vi "saltgenerator.vi"(11 "Numeric":i32) -> (3 "string":string)   [LabVIEW 2013]
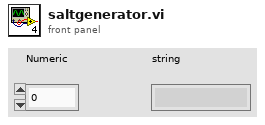
[diagram p1: front panel]
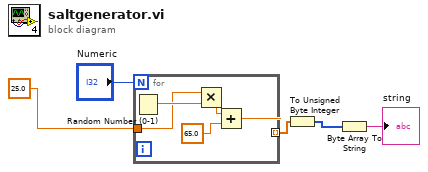
[diagram p0: block diagram]
diagram:
  n1 = for {
    N: "Numeric" -> [_]
    tunnel: 25.0 -> [w7]
    tunnel: [w6] -> w2 mode=indexing
    n2 = Random Number (0-1)() -> (number: 0 to 1=w10:dbl)
    n3 = Multiply(x=w7, y=w10) -> (x*y=w8:dbl)
    n4 = Add(x=w8, y=65.0) -> (x+y=w6:dbl)
  }
  n5 = To Unsigned Byte Integer(number=w2) -> (unsigned 8bit integer=w3:u8[])
  n6 = Byte Array To String(unsigned byte array=w3) -> (string=→"string":string)
